vi "S8300E_AskOP_PressEnter.vi"() -> ()   [LabVIEW 2011]
panel:
  in  "當看到此畫面出現才能按此button":bool
  # "2014-12-15"
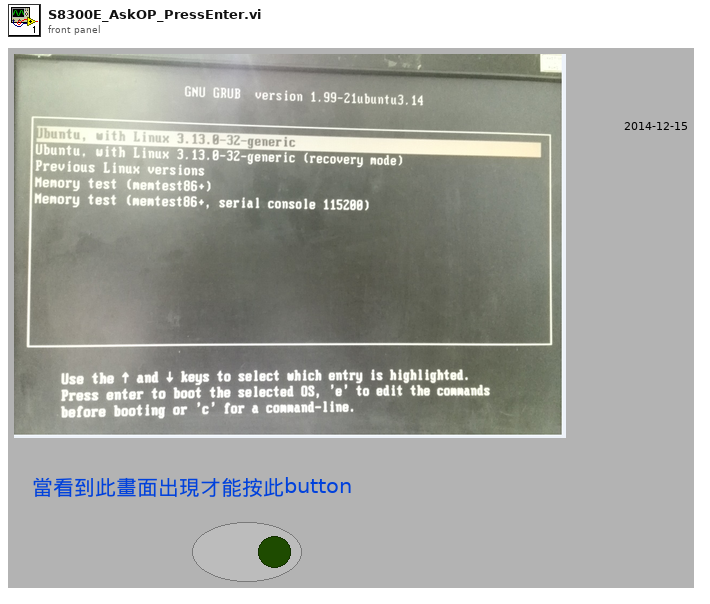
[diagram p1: front panel]
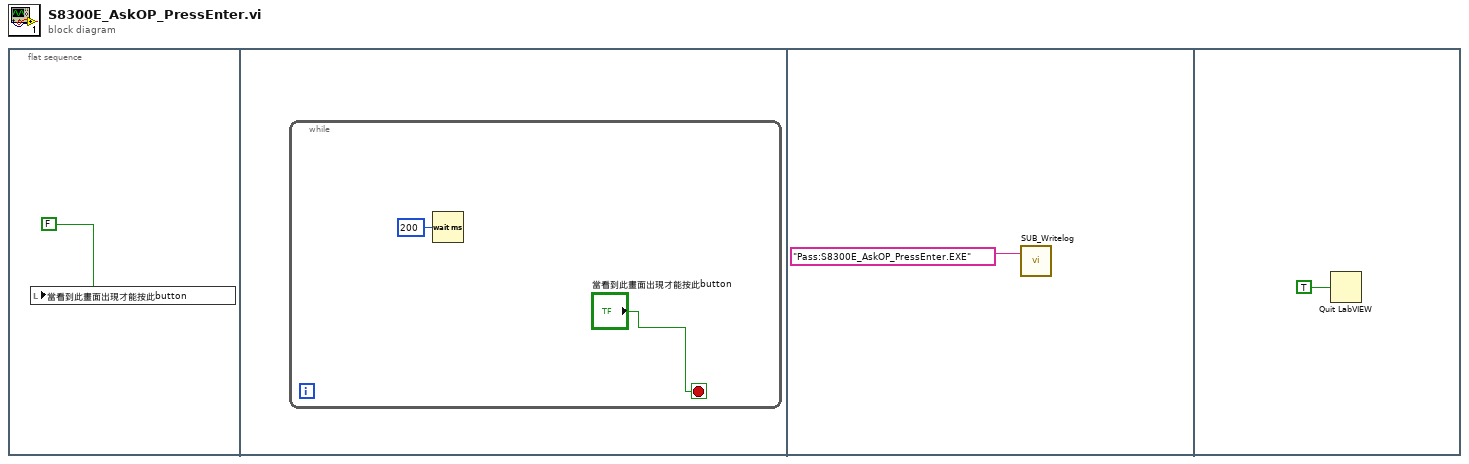
[diagram p0: block diagram]
diagram:
  n1 = flat-sequence {
    frame #0 {
      n2 = local write "當看到此畫面出現才能按此button"(FALSE) -> ()
    }
    frame #1 {
      n3 = while {
        stop <- "當看到此畫面出現才能按此button" stop-if-true
        n4 = Wait (ms)(milliseconds to wait=u32 200) -> ()  [unwired: 1 out]
      }
    }
    frame #2 {
      n5 = call "SUB_Writelog.vi"("Pass/Fail"="Pass:S8300E_AskOP_PressEnter.EXE") -> ()  [unwired: 2 in]
    }
    frame #3 {
      n6 = Quit LabVIEW(quit? (T)=TRUE) -> ()
    }
  }
